vi "WLAN - TV - RW - UTIL - StringClusterToDataType.vi"(7 "TV Paramaters(String)":T4) -> (8 "WLAN Measurement Settings":T1={"OFDM Advanced Controls(11ag)"={"OFDM Auto Compute Acquisition Length Enabled"=0, "OFDM Maximum Symbols Used"=0, "OFDM Time Tracking Enabled"=0, "OFDM Channel Tracking Enabled"=0, "OFDM Amplitude Tracking Enabled"=1, "OFDM CFO Estimation Method"=0, "OFDM Phase Tracking Method"=0, "OFDM Header Detection Enabled"=0, "OFDM MAC FCS Check Enabled"=0, "#Avg"=10, "#Iterations"=10}, "DSSS Demod Parameters"={"DSSS Auto Compute Acquisition Length Enabled"=0, "DSSS Equalization Enabled"=0, "DSSS Header Detection Enabled"=0, "DSSS MAC FCS Check Enabled"=0, "DSSS Measurement Start Location"=0, "DSSS Phase Tracking Method"=0, "DSSS Maximum Chips Used"=0, "DSSS Reference Pulse Shaping Filter"=0, "DSSS Reference Pulse Shaping Filter Coefficient"=0.0, "# Avg"=1024, "# Iterations"=1024, "DSSS Power Ramp Enabled"=0}, "OFDM Advanced Controls (11n)"={"OFDM Auto Compute Acquisition Length Enabled"=0, "OFDM Maximum Symbols Used"=0, "OFDM Time Tracking Enabled"=0, "OFDM Channel Tracking Enabled"=0, "OFDM Amplitude Tracking Enabled"=1, "OFDM CFO Estimation Method"=0, "OFDM Phase Tracking Method"=0, "OFDM Header Detection Enabled"=0, "OFDM MAC FCS Check Enabled"=0, "#Avg"=10, "#Iterations"=10}, "OFDM Advanced Controls(11ac)"={"OFDM Auto Compute Acquisition Length Enabled"=0, "OFDM Maximum Symbols Used"=0, "OFDM Time Tracking Enabled"=1, "OFDM Channel Tracking Enabled"=0, "OFDM Amplitude Tracking Enabled"=0, "OFDM CFO Estimation Method"=0, "OFDM Phase Tracking Method"=0, "OFDM Header Detection Enabled"=0, "OFDM MAC FCS Check Enabled"=0, "#Avg"=10, "#Iterations"=10}} {"OFDM Advanced Controls(11ac)"."OFDM Phase Tracking Method" items=["Standard", "Instantaneous", "None", "Standard with Cubic Spline Fit"]; "OFDM Advanced Controls(11ac)"."OFDM CFO Estimation Method" items=["Preamble Only", "Preamble and Data"]; "OFDM Advanced Controls(11ac)"."OFDM Channel Tracking Enabled" items=["False", "True"]; "OFDM Advanced Controls(11ac)"."OFDM Amplitude Tracking Enabled" items=["False", "True"]; "OFDM Advanced Controls(11ac)"."OFDM Time Tracking Enabled" items=["True"=1, "False"=0]; "OFDM Advanced Controls(11ac)"."OFDM Auto Compute Acquisition Length Enabled" items=["False", "True"]; "OFDM Advanced Controls(11ac)"."OFDM MAC FCS Check Enabled" items=["False", "True"]; "OFDM Advanced Controls(11ac)"."OFDM Header Detection Enabled" items=["False", "True"]; "OFDM Advanced Controls (11n)"."OFDM Phase Tracking Method" items=["Standard", "Instantaneous", "None", "Standard with Cubic Spline Fit"]; "OFDM Advanced Controls (11n)"."OFDM CFO Estimation Method" items=["Preamble Only", "Preamble and Data"]; "OFDM Advanced Controls (11n)"."OFDM Channel Tracking Enabled" items=["False", "True"]; "OFDM Advanced Controls (11n)"."OFDM Amplitude Tracking Enabled" items=["False", "True"]; "OFDM Advanced Controls (11n)"."OFDM Time Tracking Enabled" items=["True"=1, "False"=0]; "OFDM Advanced Controls (11n)"."OFDM Auto Compute Acquisition Length Enabled" items=["False", "True"]; "OFDM Advanced Controls (11n)"."OFDM MAC FCS Check Enabled" items=["False", "True"]; "OFDM Advanced Controls (11n)"."OFDM Header Detection Enabled" items=["False", "True"]; "DSSS Demod Parameters"."DSSS Power Ramp Enabled" items=["False", "True"]; "DSSS Demod Parameters"."DSSS Auto Compute Acquisition Length Enabled" items=["False", "True"]; "DSSS Demod Parameters"."DSSS Phase Tracking Method" items=["Standard", "Instantaneous"]; "DSSS Demod Parameters"."DSSS Equalization Enabled" items=["False", "True"]; "DSSS Demod Parameters"."DSSS Reference Pulse Shaping Filter" items=["Rectangular", "Raised Cosine", "Root Raised Cosine", "Gaussian"]; "DSSS Demod Parameters"."DSSS MAC FCS Check Enabled" items=["False", "True"]; "DSSS Demod Parameters"."DSSS Header Detection Enabled" items=["False", "True"]; "OFDM Advanced Controls(11ag)"."OFDM Phase Tracking Method" items=["Standard", "Instantaneous", "None", "Standard with Cubic Spline Fit"]; "OFDM Advanced Controls(11ag)"."OFDM CFO Estimation Method" items=["Preamble Only", "Preamble and Data"]; "OFDM Advanced Controls(11ag)"."OFDM Channel Tracking Enabled" items=["False", "True"]; "OFDM Advanced Controls(11ag)"."OFDM Amplitude Tracking Enabled" items=["False", "True"]; "OFDM Advanced Controls(11ag)"."OFDM Time Tracking Enabled" items=["True"=1, "False"=0]; "OFDM Advanced Controls(11ag)"."OFDM Auto Compute Acquisition Length Enabled" items=["False", "True"]; "OFDM Advanced Controls(11ag)"."OFDM MAC FCS Check Enabled" items=["False", "True"]; "OFDM Advanced Controls(11ag)"."OFDM Header Detection Enabled" items=["False", "True"]})   [LabVIEW 2012]
uses:
  Includes/WLAN - TV - RW - INC - Tx_Measurement_Cluster(string).ctl
  Includes/WLAN - TV - RW - INC - Tx_Meas_Settings_OFDM_String.ctl
  Includes/WLAN - TV - RW - INC - Tx_Meas_Settings_DSSS_String.ctl
  Includes/WLAN - TV - RW - INC - Tx_Measurement_Cluster.ctl
  Includes/WLAN - TV - RW - INC - TV_OFDM Demod.ctl
  Includes/WLAN - TV - RW - INC - TV_DSSS Demod.ctl
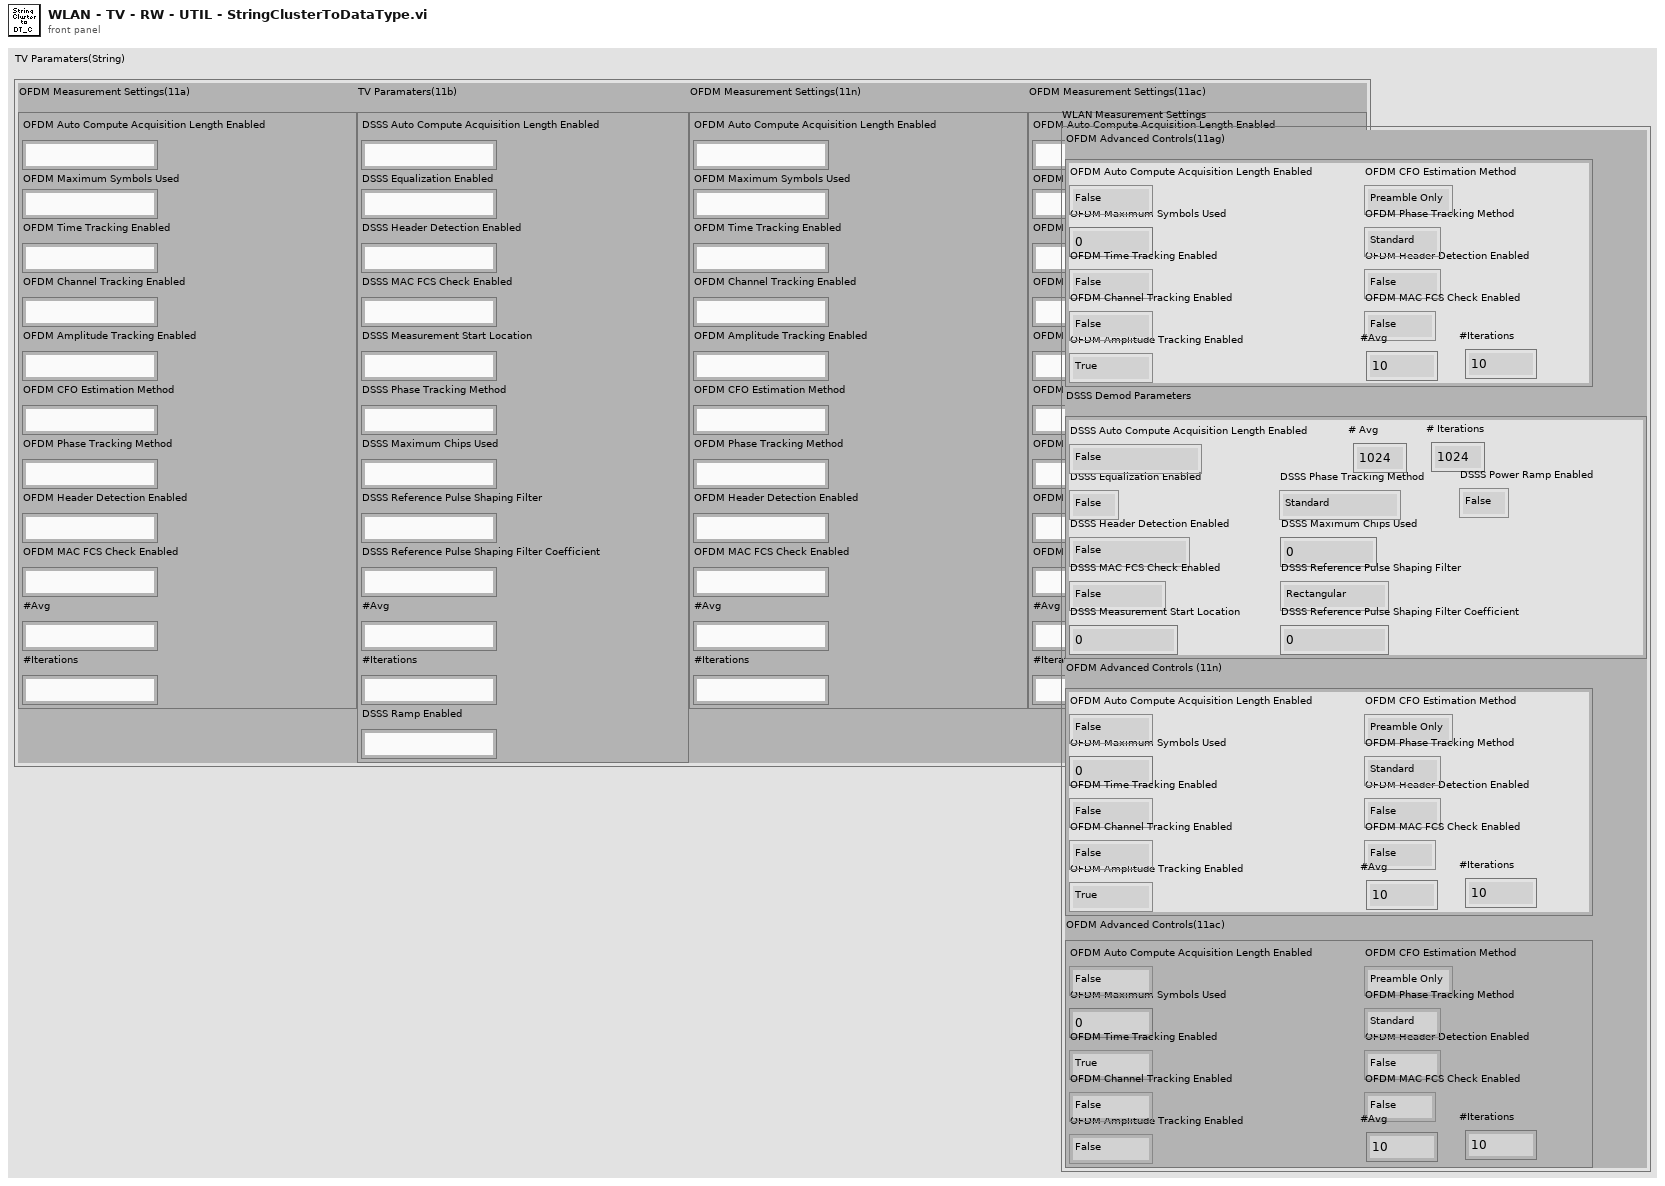
[diagram p1: front panel]
types:
  T1 = typedef "WLAN - TV - RW - INC - Tx_Measurement_Cluster.ctl" = cluster{"OFDM Advanced Controls(11ag)":T2, "DSSS Demod Parameters":T3, "OFDM Advanced Controls (11n)":T2, "OFDM Advanced Controls(11ac)":cluster{"OFDM Auto Compute Acquisition Length Enabled":i32, "OFDM Maximum Symbols Used":i32, "OFDM Time Tracking Enabled":i32, "OFDM Channel Tracking Enabled":i32, "OFDM Amplitude Tracking Enabled":i32, "OFDM CFO Estimation Method":i32, "OFDM Phase Tracking Method":i32, "OFDM Header Detection Enabled":i32, "OFDM MAC FCS Check Enabled":i32, "#Avg":i32, "#Iterations":i32}}
  T2 = typedef "WLAN - TV - RW - INC - TV_OFDM Demod.ctl" = cluster{"OFDM Auto Compute Acquisition Length Enabled":i32, "OFDM Maximum Symbols Used":i32, "OFDM Time Tracking Enabled":i32, "OFDM Channel Tracking Enabled":i32, "OFDM Amplitude Tracking Enabled":i32, "OFDM CFO Estimation Method":i32, "OFDM Phase Tracking Method":i32, "OFDM Header Detection Enabled":i32, "OFDM MAC FCS Check Enabled":i32, "#Avg":i32, "#Iterations":i32}
  T3 = typedef "WLAN - TV - RW - INC - TV_DSSS Demod.ctl" = cluster{"DSSS Auto Compute Acquisition Length Enabled":i32, "DSSS Equalization Enabled":i32, "DSSS Header Detection Enabled":i32, "DSSS MAC FCS Check Enabled":i32, "DSSS Measurement Start Location":i32, "DSSS Phase Tracking Method":i32, "DSSS Maximum Chips Used":i32, "DSSS Reference Pulse Shaping Filter":i32, "DSSS Reference Pulse Shaping Filter Coefficient":dbl, "# Avg":i32, "# Iterations":i32, "DSSS Power Ramp Enabled":i32}
  T4 = typedef "WLAN - TV - RW - INC - Tx_Measurement_Cluster(string).ctl" = cluster{"OFDM Measurement Settings(11a)":T5, "TV Paramaters(11b)":T6, "OFDM Measurement Settings(11n) ":T5, "OFDM Measurement Settings(11ac) ":T5}
  T5 = typedef "WLAN - TV - RW - INC - Tx_Meas_Settings_OFDM_String.ctl" = cluster{"OFDM Auto Compute Acquisition Length Enabled":string, "OFDM Maximum Symbols Used":string, "OFDM Time Tracking Enabled":string, "OFDM Channel Tracking Enabled":string, "OFDM Amplitude Tracking Enabled":string, "OFDM CFO Estimation Method":string, "OFDM Phase Tracking Method":string, "OFDM Header Detection Enabled":string, "OFDM MAC FCS Check Enabled":string, "#Avg":string, "#Iterations":string}
  T6 = typedef "WLAN - TV - RW - INC - Tx_Meas_Settings_DSSS_String.ctl" = cluster{"DSSS Auto Compute Acquisition Length Enabled":string, "DSSS Equalization Enabled":string, "DSSS Header Detection Enabled":string, "DSSS MAC FCS Check Enabled":string, "DSSS Measurement Start Location":string, "DSSS Phase Tracking Method":string, "DSSS Maximum Chips Used":string, "DSSS Reference Pulse Shaping Filter":string, "DSSS Reference Pulse Shaping Filter Coefficient":string, "#Avg":string, "#Iterations":string, "DSSS Ramp Enabled ":string}
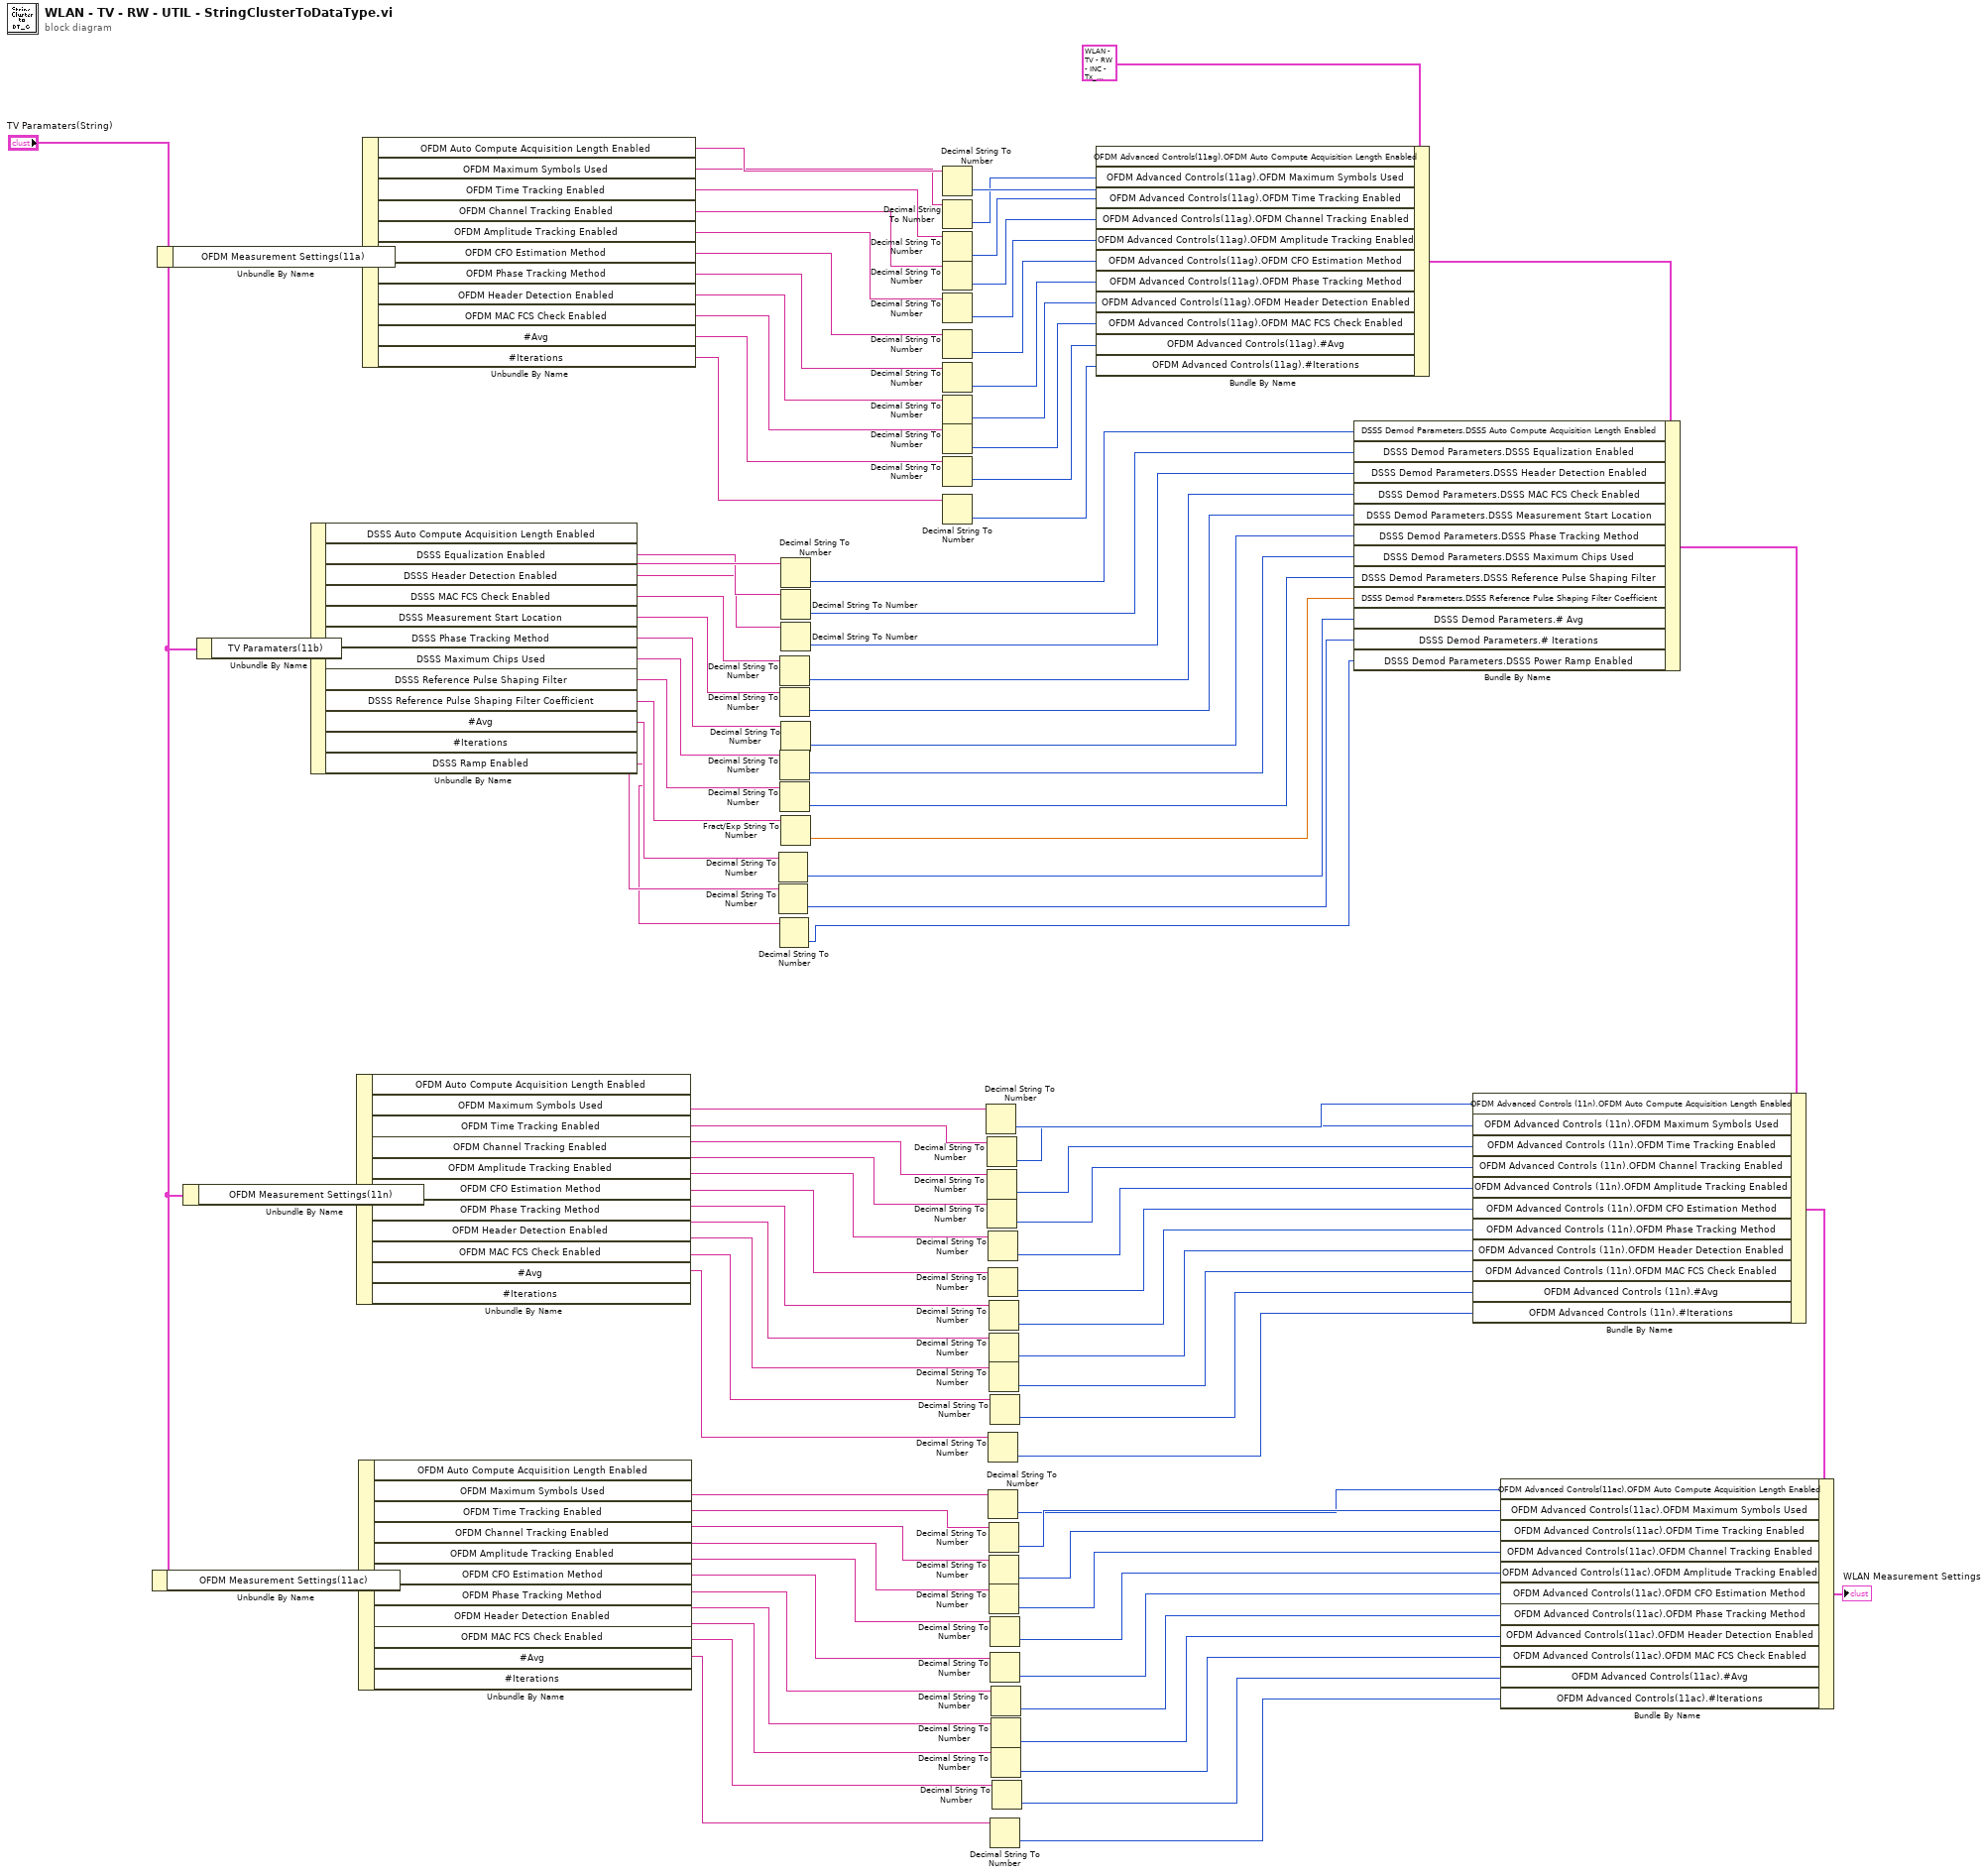
[diagram p0: block diagram]
diagram:
  n1 = Unbundle By Name("TV Paramaters(String)") -> ("OFDM Measurement Settings(11ac)"=w3:T5)
  n2 = Unbundle By Name("TV Paramaters(String)") -> ("OFDM Measurement Settings(11a)"=w4:T5)
  n3 = Unbundle By Name("TV Paramaters(String)") -> ("OFDM Measurement Settings(11n)"=w6:T5)
  n4 = Unbundle By Name("TV Paramaters(String)") -> ("TV Paramaters(11b)"=w2:T6)
  n5 = Unbundle By Name(w2) -> ("DSSS Auto Compute Acquisition Length Enabled"=w100:string, "DSSS Equalization Enabled"=w99:string, "DSSS Header Detection Enabled"=w98:string, "DSSS MAC FCS Check Enabled"=w97:string, "DSSS Measurement Start Location"=w96:string, "DSSS Phase Tracking Method"=w34:string, "DSSS Maximum Chips Used"=w95:string, "DSSS Reference Pulse Shaping Filter"=w94:string, "DSSS Reference Pulse Shaping Filter Coefficient"=w35:string, "#Avg"=w93:string, "#Iterations"=w92:string, "DSSS Ramp Enabled"=w7:string)
  n6 = Unbundle By Name(w6) -> ("OFDM Auto Compute Acquisition Length Enabled"=w80:string, "OFDM Maximum Symbols Used"=w79:string, "OFDM Time Tracking Enabled"=w78:string, "OFDM Channel Tracking Enabled"=w77:string, "OFDM Amplitude Tracking Enabled"=w76:string, "OFDM CFO Estimation Method"=w75:string, "OFDM Phase Tracking Method"=w74:string, "OFDM Header Detection Enabled"=w73:string, "OFDM MAC FCS Check Enabled"=w72:string, "#Avg"=w71:string, "#Iterations"=w70:string)
  n7 = Unbundle By Name(w3) -> ("OFDM Auto Compute Acquisition Length Enabled"=w10:string, "OFDM Maximum Symbols Used"=w11:string, "OFDM Time Tracking Enabled"=w12:string, "OFDM Channel Tracking Enabled"=w13:string, "OFDM Amplitude Tracking Enabled"=w14:string, "OFDM CFO Estimation Method"=w15:string, "OFDM Phase Tracking Method"=w16:string, "OFDM Header Detection Enabled"=w17:string, "OFDM MAC FCS Check Enabled"=w18:string, "#Avg"=w19:string, "#Iterations"=w20:string)
  n8 = Unbundle By Name(w4) -> ("OFDM Auto Compute Acquisition Length Enabled"=w91:string, "OFDM Maximum Symbols Used"=w90:string, "OFDM Time Tracking Enabled"=w89:string, "OFDM Channel Tracking Enabled"=w88:string, "OFDM Amplitude Tracking Enabled"=w87:string, "OFDM CFO Estimation Method"=w86:string, "OFDM Phase Tracking Method"=w85:string, "OFDM Header Detection Enabled"=w84:string, "OFDM MAC FCS Check Enabled"=w83:string, "#Avg"=w82:string, "#Iterations"=w81:string)
  n9 = Decimal String To Number(string=w93) -> (number=w55:i32)  [unwired: 2 in, 1 out]
  n10 = Decimal String To Number(string=w92) -> (number=w56:i32)  [unwired: 2 in, 1 out]
  n11 = Decimal String To Number(string=w7) -> (number=w1:i32)  [unwired: 2 in, 1 out]
  n12 = Decimal String To Number(string=w97) -> (number=w51:i32)  [unwired: 2 in, 1 out]
  n13 = Decimal String To Number(string=w96) -> (number=w52:i32)  [unwired: 2 in, 1 out]
  n14 = Decimal String To Number(string=w95) -> (number=w53:i32)  [unwired: 2 in, 1 out]
  n15 = Decimal String To Number(string=w94) -> (number=w54:i32)  [unwired: 2 in, 1 out]
  n16 = Decimal String To Number(string=w100) -> (number=w48:i32)  [unwired: 2 in, 1 out]
  n17 = Decimal String To Number(string=w99) -> (number=w49:i32)  [unwired: 2 in, 1 out]
  n18 = Decimal String To Number(string=w98) -> (number=w50:i32)  [unwired: 2 in, 1 out]
  n19 = Decimal String To Number(string=w34) -> (number=w33:i32)  [unwired: 2 in, 1 out]
  n20 = Fract/Exp String To Number(string=w35) -> (number=w32:dbl)  [unwired: 3 in, 1 out]
  n21 = Decimal String To Number(string=w91) -> (number=w69:i32)  [unwired: 2 in, 1 out]
  n22 = Decimal String To Number(string=w90) -> (number=w67:i32)  [unwired: 2 in, 1 out]
  n23 = Decimal String To Number(string=w89) -> (number=w68:i32)  [unwired: 2 in, 1 out]
  n24 = Decimal String To Number(string=w88) -> (number=w65:i32)  [unwired: 2 in, 1 out]
  n25 = Decimal String To Number(string=w87) -> (number=w66:i32)  [unwired: 2 in, 1 out]
  n26 = Decimal String To Number(string=w86) -> (number=w64:i32)  [unwired: 2 in, 1 out]
  n27 = Decimal String To Number(string=w85) -> (number=w63:i32)  [unwired: 2 in, 1 out]
  n28 = Decimal String To Number(string=w84) -> (number=w62:i32)  [unwired: 2 in, 1 out]
  n29 = Decimal String To Number(string=w83) -> (number=w61:i32)  [unwired: 2 in, 1 out]
  n30 = Decimal String To Number(string=w82) -> (number=w60:i32)  [unwired: 2 in, 1 out]
  n31 = Decimal String To Number(string=w81) -> (number=w59:i32)  [unwired: 2 in, 1 out]
  n32 = Decimal String To Number(string=w80) -> (number=w46:i32)  [unwired: 2 in, 1 out]
  n33 = Decimal String To Number(string=w79) -> (number=w36:i32)  [unwired: 2 in, 1 out]
  n34 = Decimal String To Number(string=w78) -> (number=w37:i32)  [unwired: 2 in, 1 out]
  n35 = Decimal String To Number(string=w77) -> (number=w38:i32)  [unwired: 2 in, 1 out]
  n36 = Decimal String To Number(string=w76) -> (number=w39:i32)  [unwired: 2 in, 1 out]
  n37 = Decimal String To Number(string=w75) -> (number=w40:i32)  [unwired: 2 in, 1 out]
  n38 = Decimal String To Number(string=w70) -> (number=w45:i32)  [unwired: 2 in, 1 out]
  n39 = Decimal String To Number(string=w10) -> (number=w21:i32)  [unwired: 2 in, 1 out]
  n40 = Decimal String To Number(string=w74) -> (number=w41:i32)  [unwired: 2 in, 1 out]
  n41 = Decimal String To Number(string=w73) -> (number=w42:i32)  [unwired: 2 in, 1 out]
  n42 = Decimal String To Number(string=w72) -> (number=w43:i32)  [unwired: 2 in, 1 out]
  n43 = Decimal String To Number(string=w11) -> (number=w31:i32)  [unwired: 2 in, 1 out]
  n44 = Decimal String To Number(string=w12) -> (number=w30:i32)  [unwired: 2 in, 1 out]
  n45 = Decimal String To Number(string=w13) -> (number=w29:i32)  [unwired: 2 in, 1 out]
  n46 = Decimal String To Number(string=w71) -> (number=w44:i32)  [unwired: 2 in, 1 out]
  n47 = Decimal String To Number(string=w14) -> (number=w28:i32)  [unwired: 2 in, 1 out]
  n48 = Decimal String To Number(string=w15) -> (number=w27:i32)  [unwired: 2 in, 1 out]
  n49 = Decimal String To Number(string=w20) -> (number=w22:i32)  [unwired: 2 in, 1 out]
  n50 = Decimal String To Number(string=w16) -> (number=w26:i32)  [unwired: 2 in, 1 out]
  n51 = Decimal String To Number(string=w17) -> (number=w25:i32)  [unwired: 2 in, 1 out]
  n52 = Decimal String To Number(string=w18) -> (number=w24:i32)  [unwired: 2 in, 1 out]
  n53 = Decimal String To Number(string=w19) -> (number=w23:i32)  [unwired: 2 in, 1 out]
  n54 = Bundle By Name(cluster=T1 {"OFDM Advanced Controls(11ag)"={"OFDM Auto Compute Acquisition Length Enabled"=0, "OFDM Maximum Symbols Used"=0, "OFDM Time Tracking Enabled"=0, "OFDM Channel Tracking Enabled"=0, "OFDM Amplitude Tracking Enabled"=1, "OFDM CFO Estimation Method"=0, "OFDM Phase Tracking Method"=0, "OFDM Header Detection Enabled"=0, "OFDM MAC FCS Check Enabled"=0, "#Avg"=10, "#Iterations"=10}, "DSSS Demod Parameters"={"DSSS Auto Compute Acquisition Length Enabled"=0, "DSSS Equalization Enabled"=0, "DSSS Header Detection Enabled"=0, "DSSS MAC FCS Check Enabled"=0, "DSSS Measurement Start Location"=0, "DSSS Phase Tracking Method"=0, "DSSS Maximum Chips Used"=0, "DSSS Reference Pulse Shaping Filter"=0, "DSSS Reference Pulse Shaping Filter Coefficient"=0.0, "# Avg"=1024, "# Iterations"=1024, "DSSS Power Ramp Enabled"=0}, "OFDM Advanced Controls (11n)"={"OFDM Auto Compute Acquisition Length Enabled"=0, "OFDM Maximum Symbols Used"=0, "OFDM Time Tracking Enabled"=0, "OFDM Channel Tracking Enabled"=0, "OFDM Amplitude Tracking Enabled"=1, "OFDM CFO Estimation Method"=0, "OFDM Phase Tracking Method"=0, "OFDM Header Detection Enabled"=0, "OFDM MAC FCS Check Enabled"=0, "#Avg"=10, "#Iterations"=10}, "OFDM Advanced Controls(11ac)"={"OFDM Auto Compute Acquisition Length Enabled"=0, "OFDM Maximum Symbols Used"=0, "OFDM Time Tracking Enabled"=0, "OFDM Channel Tracking Enabled"=0, "OFDM Amplitude Tracking Enabled"=0, "OFDM CFO Estimation Method"=0, "OFDM Phase Tracking Method"=0, "OFDM Header Detection Enabled"=0, "OFDM MAC FCS Check Enabled"=0, "#Avg"=0, "#Iterations"=0}} ("WLAN Measurement Settings"), "OFDM Advanced Controls(11ag).OFDM Auto Compute Acquisition Length Enabled"=w69, "OFDM Advanced Controls(11ag).OFDM Maximum Symbols Used"=w67, "OFDM Advanced Controls(11ag).OFDM Time Tracking Enabled"=w68, "OFDM Advanced Controls(11ag).OFDM Channel Tracking Enabled"=w65, "OFDM Advanced Controls(11ag).OFDM Amplitude Tracking Enabled"=w66, "OFDM Advanced Controls(11ag).OFDM CFO Estimation Method"=w64, "OFDM Advanced Controls(11ag).OFDM Phase Tracking Method"=w63, "OFDM Advanced Controls(11ag).OFDM Header Detection Enabled"=w62, "OFDM Advanced Controls(11ag).OFDM MAC FCS Check Enabled"=w61, "OFDM Advanced Controls(11ag).#Avg"=w60, "OFDM Advanced Controls(11ag).#Iterations"=w59) -> (w57:T1)
  n55 = Bundle By Name(cluster=w57, "DSSS Demod Parameters.DSSS Auto Compute Acquisition Length Enabled"=w48, "DSSS Demod Parameters.DSSS Equalization Enabled"=w49, "DSSS Demod Parameters.DSSS Header Detection Enabled"=w50, "DSSS Demod Parameters.DSSS MAC FCS Check Enabled"=w51, "DSSS Demod Parameters.DSSS Measurement Start Location"=w52, "DSSS Demod Parameters.DSSS Phase Tracking Method"=w33, "DSSS Demod Parameters.DSSS Maximum Chips Used"=w53, "DSSS Demod Parameters.DSSS Reference Pulse Shaping Filter"=w54, "DSSS Demod Parameters.DSSS Reference Pulse Shaping Filter Coefficient"=w32, "DSSS Demod Parameters.# Avg"=w55, "DSSS Demod Parameters.# Iterations"=w56, "DSSS Demod Parameters.DSSS Power Ramp Enabled"=w1) -> (w47:T1)
  n56 = Bundle By Name(cluster=w47, "OFDM Advanced Controls (11n).OFDM Auto Compute Acquisition Length Enabled"=w46, "OFDM Advanced Controls (11n).OFDM Maximum Symbols Used"=w36, "OFDM Advanced Controls (11n).OFDM Time Tracking Enabled"=w37, "OFDM Advanced Controls (11n).OFDM Channel Tracking Enabled"=w38, "OFDM Advanced Controls (11n).OFDM Amplitude Tracking Enabled"=w39, "OFDM Advanced Controls (11n).OFDM CFO Estimation Method"=w40, "OFDM Advanced Controls (11n).OFDM Phase Tracking Method"=w41, "OFDM Advanced Controls (11n).OFDM Header Detection Enabled"=w42, "OFDM Advanced Controls (11n).OFDM MAC FCS Check Enabled"=w43, "OFDM Advanced Controls (11n).#Avg"=w44, "OFDM Advanced Controls (11n).#Iterations"=w45) -> (w9:T1)
  n57 = Bundle By Name(cluster=w9, "OFDM Advanced Controls(11ac).OFDM Auto Compute Acquisition Length Enabled"=w21, "OFDM Advanced Controls(11ac).OFDM Maximum Symbols Used"=w31, "OFDM Advanced Controls(11ac).OFDM Time Tracking Enabled"=w30, "OFDM Advanced Controls(11ac).OFDM Channel Tracking Enabled"=w29, "OFDM Advanced Controls(11ac).OFDM Amplitude Tracking Enabled"=w28, "OFDM Advanced Controls(11ac).OFDM CFO Estimation Method"=w27, "OFDM Advanced Controls(11ac).OFDM Phase Tracking Method"=w26, "OFDM Advanced Controls(11ac).OFDM Header Detection Enabled"=w25, "OFDM Advanced Controls(11ac).OFDM MAC FCS Check Enabled"=w24, "OFDM Advanced Controls(11ac).#Avg"=w23, "OFDM Advanced Controls(11ac).#Iterations"=w22) -> (→"WLAN Measurement Settings":T1)
